vi "Open Connection_command_exitControl.vi"(8 "error in (no error)":errorcluster, 9 "command_exitControl":T1, 10 "topicName":string) -> (0 "error out":errorcluster, 3 "topicRef":cluster{"topicName":string, "type":refnum<vi>})   [LabVIEW 2015]
uses:
  SALTypedefs/m2ms/command_exitControl.ctl
  SALTypedefs/m2ms/m2ms.lvlib
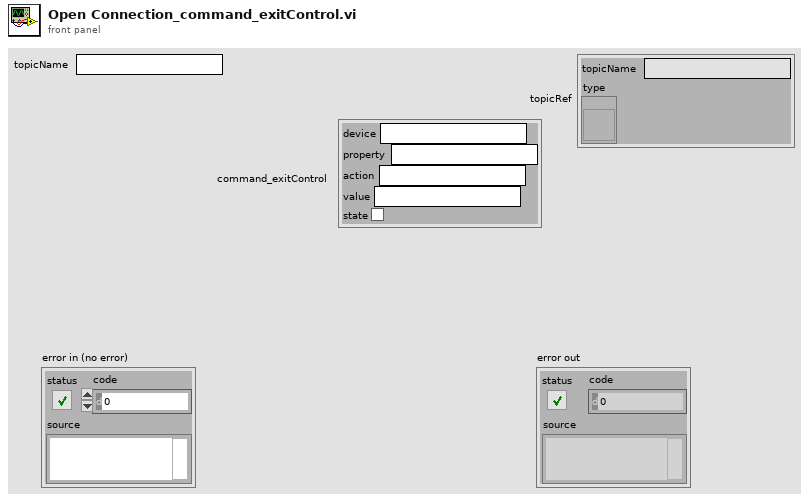
[diagram p1: front panel]
types:
  T1 = typedef "m2ms.lvlib/command_exitControl.ctl" = cluster{"device":string, "property":string, "action":string, "value":string, "state":bool}
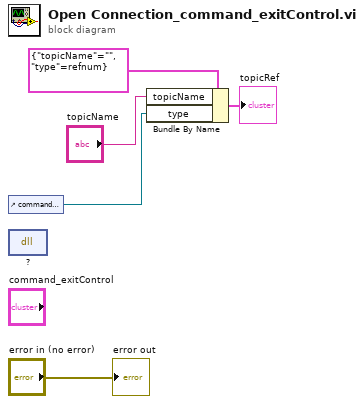
[diagram p0: block diagram]
diagram:
  n1 = control-ref of="command_exitControl"() -> (w2:refnum<vi>)
  n2 = dll-call lib="?" fn="?"() -> ()  [unwired: 4 in, 2 out]
  n3 = Bundle By Name(cluster=cluster{"topicName":string, "type":refnum<vi>} {"topicName"="", "type"=refnum} ("topicRef"), "topicName"="topicName", "type"=w2) -> (→"topicRef":cluster{"topicName":string, "type":refnum<vi>})
  "error out" <- "error in (no error)"
